vi "set voltage.vi"(8 "error in (no error)":errorcluster, 10 "Voltage":dbl, 11 "PSP-603 in":refnum<class "PSP-603.lvclass">) -> (0 "error out":errorcluster, 3 "PSP-603 out":refnum<class "PSP-603.lvclass">)   [LabVIEW 2025, in "Power Supply.lvlib" / "PSP-603.lvclass"]
uses:
  PSP-603.lvclass
  PSP-603.lvclass/PSP-603.ctl
panel:
  out "concatenated string":string
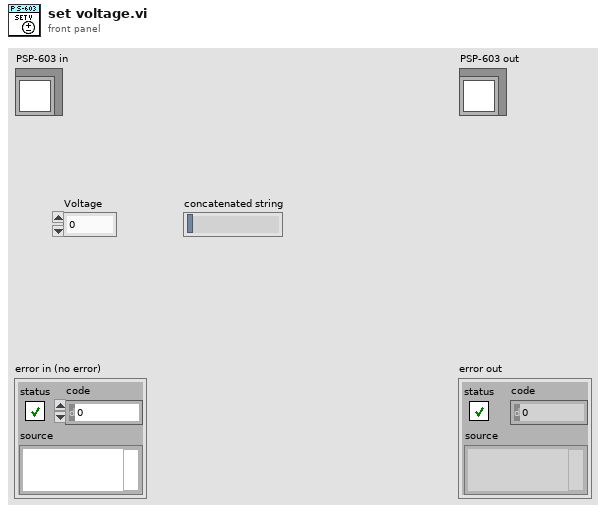
[diagram p1: front panel]
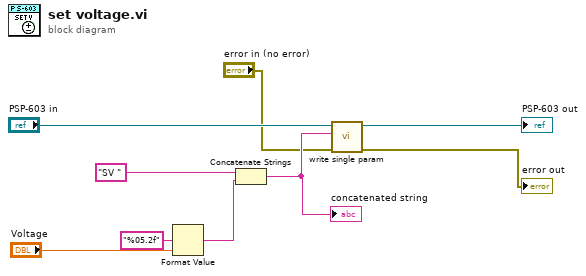
[diagram p0: block diagram]
diagram:
  n1 = Format Value(format string="%05.2f", value (0)="Voltage") -> (output string=w4:string)  [unwired: 1 in]
  n2 = Concatenate Strings("SV ", w4) -> (w3:string)
  "concatenated string" <- w3
  n3 = call-dynamic "write single param.vi"("error in (no error)"="error in (no error)", "string"=w3, "PSP-603 in"="PSP-603 in") -> ("error out"=→"error out":errorcluster, "PSP-603 out"=→"PSP-603 out":refnum<class "PSP-603.lvclass">)  [unwired: 7 in]
